vi "checkMotorLimits.vi"(11 "Device in":refnum<k24>) -> (0 "Motor Limits":bool, 3 "Device out":refnum<k24>)   [LabVIEW 2014]
uses:
  C:/user-Lab/AndreTec/GITs/andretec/Thorlabs-Vector-Move/kinesisTec/Kinesis/Thorlabs.MotionControl.TCube.DCServoCLI.dll
  kinesisTec/Kinesis/Thorlabs.MotionControl.TCube.DCServoCLI.dll
  C:/user-Lab/AndreTec/GITs/andretec/Thorlabs-Vector-Move/kinesisTec/Kinesis/Thorlabs.MotionControl.GenericMotorCLI.dll
  kinesisTec/Kinesis/Thorlabs.MotionControl.GenericMotorCLI.dll
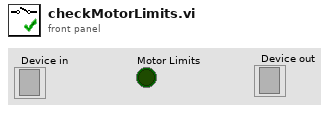
[diagram p1: front panel]
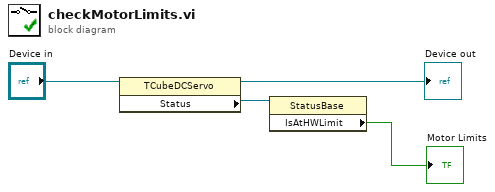
[diagram p0: block diagram]
diagram:
  n1 = property class="TCubeDCServo"(reference="Device in") -> (reference out=→"Device out":refnum<k24>, "Status"=w3:refnum<k24>)  [unwired: 1 in, 1 out]
  n2 = property class="StatusBase"(reference=w3) -> ("IsAtHWLimit"=→"Motor Limits":bool)  [unwired: 1 in, 2 out]
